vi "Pack Step Value.vi"(8 "error in (no error)":errorcluster, 10 "Value":string, 11 "DBL STEP in":refnum<class "DBL STEP.lvclass">) -> (0 "error out":errorcluster, 3 "DBL STEP out":refnum<class "DBL STEP.lvclass">)   [LabVIEW 2014, in "DBL STEP.lvlib" / "DBL STEP.lvclass"]
uses:
  DBL STEP.lvclass
  DBL STEP.lvclass/DBL STEP.ctl
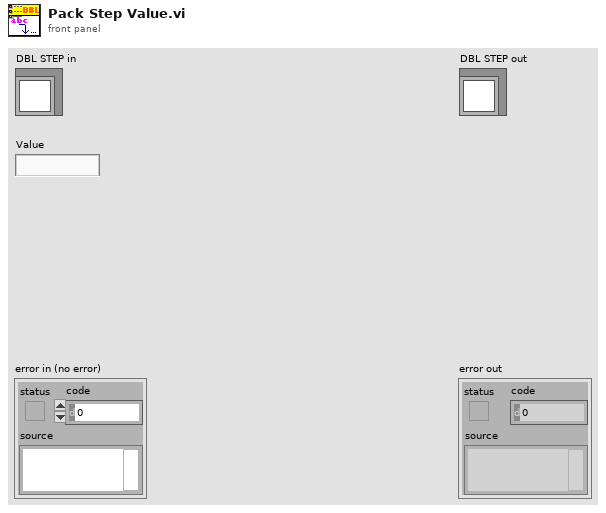
[diagram p1: front panel]
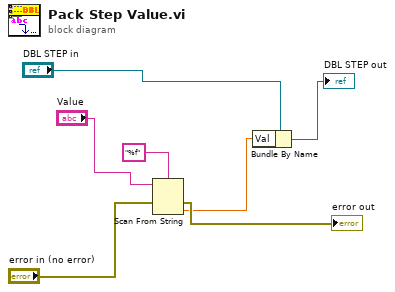
[diagram p0: block diagram]
diagram:
  n1 = Scan From String(format string="%f", input string="Value", error in="error in (no error)") -> (error out=→"error out":errorcluster, output 1=w1:dbl)  [unwired: 2 in, 2 out]
  n2 = Bundle By Name(cluster="DBL STEP in", "Val"=w1) -> (→"DBL STEP out":refnum<class "DBL STEP.lvclass">)
